vi "ULxTemperature.vi"() -> (0 "Temperature":dbl)   [LabVIEW 2016]
doc: "I. Description:\nThis example demonstrates how to make temperature measurement using a thermocouple.\n\nII. Instructions for Running:\nSpecify the Physical Channel where your signal is input on the DAQ device.\n\n\nIII. Block Diagram Steps:\n1. Create a temperature measurement channel.\n2. Call the Read VI to read one point of data.\n3. Call the Clear Task VI to clear the Task \n4. Use the popup dialog box to display an error if any.\n\nIV. I/O Connections Overview:\nConnect your thermocouple to the terminals corresponding to the Physical Channel I/O Control value."
uses:
  <vilib>/Utility/error.llb/DialogType.ctl
  <vilib>/ULx/Create Channel.llb/ULx Create Channel (AI-Temperature).vi
  <vilib>/ULx/Read.llb/ULx Read (Analog DBL 1Chan 1Samp).vi
panel:
  in  "Physical Channel":refnum<k21>="Dev0/Ti3"
  in  "Units":i32(ring)=2 items=["DegC"=0, "DegF"=1, "Kelvins"=2, "Volts"=4, "Raw"=5]
  # "Channel Parameters"
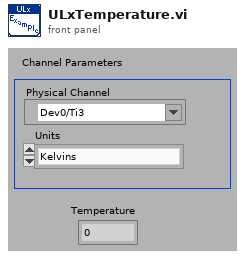
[diagram p1: front panel]
types:
  T1 = typedef "DialogType.ctl" = u16
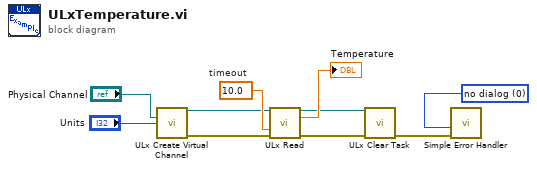
[diagram p0: block diagram]
diagram:
  w7 = T1 0 items=["no dialog", "OK message", "continue or stop message", "OK message + warnings", "continue/stop + warnings"] ("type of dialog (OK msg:1)")
  w8 = 10.0  # timeout
  n1 = call-poly <vilib>:"ULx Create Virtual Channel.vi"("physical channels"="Physical Channel", "units"="Units") -> ("task out"=w2:refnum<k24>, "error out"=w10:errorcluster)  [unwired: 12 in]
  n2 = call-poly <vilib>:"ULx Read.vi"("task in"=w2, "timeout"=w8, "error in"=w10) -> ("task out"=w6:refnum<k24>, "data"=→"Temperature":dbl, "error out"=w5:errorcluster)  [unwired: 10 in]
  n3 = call <vilib>:"ULx Clear Task.vi"("task in"=w6, "error in"=w5) -> ("error out"=w4:errorcluster)  [unwired: 13 in]
  n4 = call <vilib>:"Simple Error Handler.vi"("type of dialog (OK msg:1)"=w7, "error in (no error)"=w4) -> ()  [unwired: 3 in, 5 out]
